vi "CSMExampleBrowser_Change Bookmark Image.vi"(7 "Picture Control Reference":refnum<vi>, 8 "error in (no error)":errorcluster, 9 "No Image?":bool, 10 "Bookmark ID":u32, 11 "vi path":path) -> (0 "error out":errorcluster)   [LabVIEW 2017]
uses:
  <vilib>/Utility/miscctls.llb/LVPointTypeDef.ctl
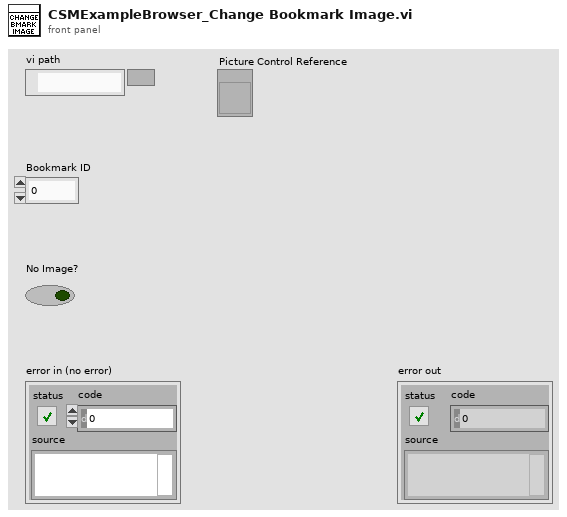
[diagram p1: front panel]
types:
  T1 = typedef "LVPointTypeDef.ctl" = cluster{"Horizontal":i16, "Vertical":i16}
  T2 = cluster{"horizontal":enum16{"left", "center", "right"}, "vertical":enum16{"top", "center", "bottom"}}
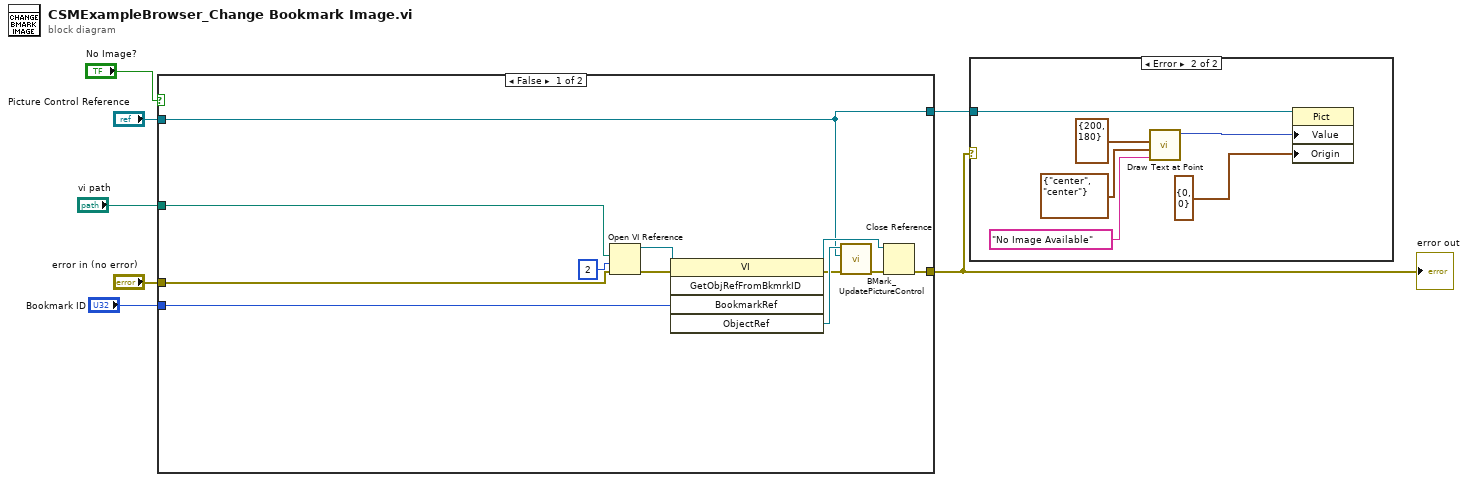
[diagram p0: block diagram]
diagram:
  n1 = case shown="False" "No Image?" {
    tunnel: [w19 w21] -> w2
    tunnel: "error in (no error)" -> [w15 w21]
    tunnel: "Picture Control Reference" -> [w8 w20]
    tunnel: "Bookmark ID" -> [w10 _]
    tunnel: "vi path" -> [w9 _]
    tunnel: [w8 w20] -> w1
    frame False {
      n2 = Open VI Reference(vi path=w9, options=2, error in (no error)=w15) -> (vi reference=w17:refnum<vi>, error out=w18:errorcluster)  [unwired: 3 in]
      n3 = invoke class="VI" method="GetObjRefFromBkmrkID"(reference=w17, error in=w18, "BookmarkRef"=w10) -> (reference out=w16:refnum<vi>, error out=w12:errorcluster, "ObjectRef"=w14:refnum<vi>)  [unwired: 2 in, 2 out]
      n4 = call "BMark_UpdatePictureControl.vi"("error in (no error)"=w12, "Picture Control Reference"=w8, "Center Object Reference"=w14) -> ("error out"=w13:errorcluster)  [unwired: 8 in]
      n5 = Close Reference(reference=w16, error in (no error)=w13) -> (error out=w19:errorcluster)
    }
    frame True {
    }
  }
  "error out" <- w2
  n6 = case shown="Error" w2 {
    tunnel: w1 -> [_ w22]
    frame No Error {
    }
    frame Error {
      n7 = call <vilib>:"Draw Text at Point.vi"("text"="No Image Available", "alignment(left, top)"=T2 {"horizontal"=enum."center", "vertical"=enum."center"}, "origin"=cluster{"x":i16, "y":i16} {"x"=200, "y"=180}) -> ("new picture"=w27:picture)  [unwired: 7 in, 1 out]
      n8 = property class="Pict"(reference=w22, "Value"=w27, "Origin"=T1 {"Horizontal"=0, "Vertical"=0}) -> ()  [unwired: 1 in, 2 out]
    }
  }
